vi "Set ASCII Precision.vi"(0 "VISA resource name":refnum<visa-resource-name>, 9 "ASCII Precision Digits":i16=6 min=0 max=16, 11 "error in (no error)":errorcluster) -> (4 "VISA resource name out":refnum<visa-resource-name>, 15 "error Out (no error)":errorcluster)   [LabVIEW 2018, in "Keithley DMM7512.lvlib"]
doc: "This VI sets the precision (number of digits) for all numbers returned in the ASCII format."
uses:
  <instrlib>/Keithley DMM7512/Keithley DMM7512.lvlib
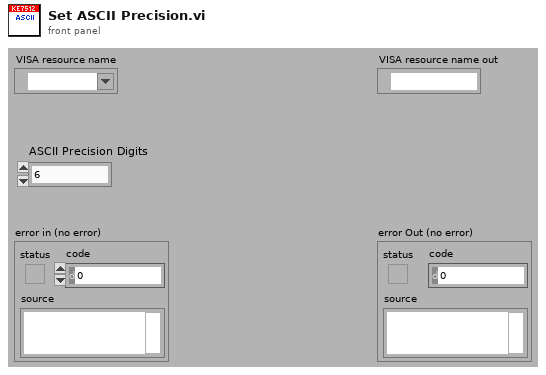
[diagram p1: front panel]
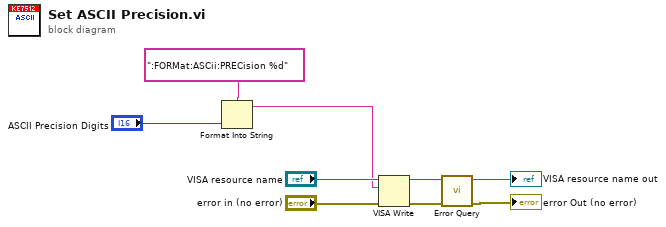
[diagram p0: block diagram]
diagram:
  n1 = Format Into String(format string=":FORMat:ASCii:PRECision %d", "ASCII Precision Digits") -> (resulting string=w5:string)  [unwired: 2 in, 1 out]
  n2 = VISA Write(VISA resource name="VISA resource name", write buffer=w5, error in (no error)="error in (no error)") -> (VISA resource name out=w4:refnum<visa-resource-name>, error out=w3:errorcluster)  [unwired: 1 out]
  n3 = call <instrlib>:"Error Query.vi"("error in (no error)"=w3, "VISA resource name"=w4) -> ("error out"=→"error Out (no error)":errorcluster, "VISA resource name out"=→"VISA resource name out":refnum<visa-resource-name>)  [unwired: 6 in, 2 out]
